vi "Find Elements not On Other Child.vi"(10 "Schedule":u16[](array[numeric]), 11 "Sub Array":u16[](array[numeric])) -> (3 "Elements to append":i32[](array[numeric]))   [LabVIEW 2013, in "GA.lvclass"]
uses:
  GA.lvclass
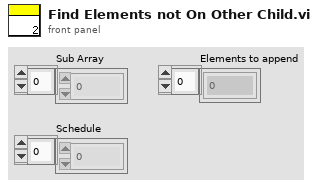
[diagram p1: front panel]
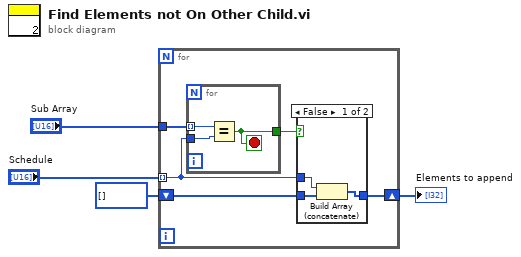
[diagram p0: block diagram]
diagram:
  n1 = for {
    tunnel: "Schedule" -> [w5] mode=indexing
    tunnel: "Sub Array" -> [w9]
    shift-right: [w6] -> w1
    shift-left: i32[] [] -> [w7]
    n2 = for {
      tunnel: w9 -> [w16] mode=indexing
      tunnel: w5 -> [w14]
      tunnel: [w15] -> w8
      stop <- w15 stop-if-true
      n3 = Equal?(x=w16, y=w14) -> (x = y?=w15:bool)
    }
    n4 = case shown="False" w8 {
      tunnel: w7 -> [w11 w13]
      tunnel: [w10 w13] -> w6
      tunnel: w5 -> [w12 _]
      frame False {
        n5 = Build Array (concatenate)(w12, w11) -> (w10:i32[])
      }
      frame True {
      }
    }
  }
  "Elements to append" <- w1
